vi "Get All Data Channels.vi"(8 "error in (no error)":errorcluster, 10 "framework configuration in":T1, 11 "VeriStand Data Sharing Framework in":refnum<class "VeriStand DSF.lvclass">) -> (0 "error out":errorcluster, 2 "data channel offsets":u64[](array[numeric]) format="%.0x", 3 "VeriStand Data Sharing Framework out":refnum<class "VeriStand DSF.lvclass">)   [LabVIEW 2017, in "DSF Engine.lvlib" / "VeriStand DSF.lvclass"]
uses:
  VeriStand DSF.lvclass
  DSF Core.lvlibp/Typedefs/DSF Engine Framework Configuration.ctl
  DSF Core.lvlibp/Typedefs/DSF Engine Plugin Configuration.ctl
  DSF Core.lvlibp/Typedefs/DSF Timing Info.ctl
  DSF Core.lvlibp/Typedefs/DSF Engine Plugin Thread Configuration.ctl
  DSF Core.lvlibp/Typedefs/DSF Settings Info.ctl
  DSF Core.lvlibp/Typedefs/DSF Engine Transfer Group Configuration.ctl
  DSF Core.lvlibp/Typedefs/DSF Direction.ctl
  DSF Core.lvlibp/Typedefs/DSF Engine Transfer Configuration.ctl
  DSF Core.lvlibp/Typedefs/DSF Byte Order.ctl
  DSF Core.lvlibp/Typedefs/DSF Engine Channel Configuration.ctl
  DSF Core.lvlibp/Typedefs/DSF Data Type.ctl
  DSF Core.lvlibp/Typedefs/DSF Timeout Behavior.ctl
  VeriStand DSF.lvclass/VeriStand DSF.ctl
  <vilib>/NI Veristand/Custom Device API/Data Access Type.ctl
  DSF Core.lvlibp/Classes/Configuration/Channel Count (Transfer).vi
  <vilib>/NI Veristand/Custom Device API/Custom Device API.lvlib
  DSF Core.lvlibp
  DSF Core.lvlibp/Classes/Configuration/Configuration Session.lvclass
  Shared/DSF Shared.lvlib
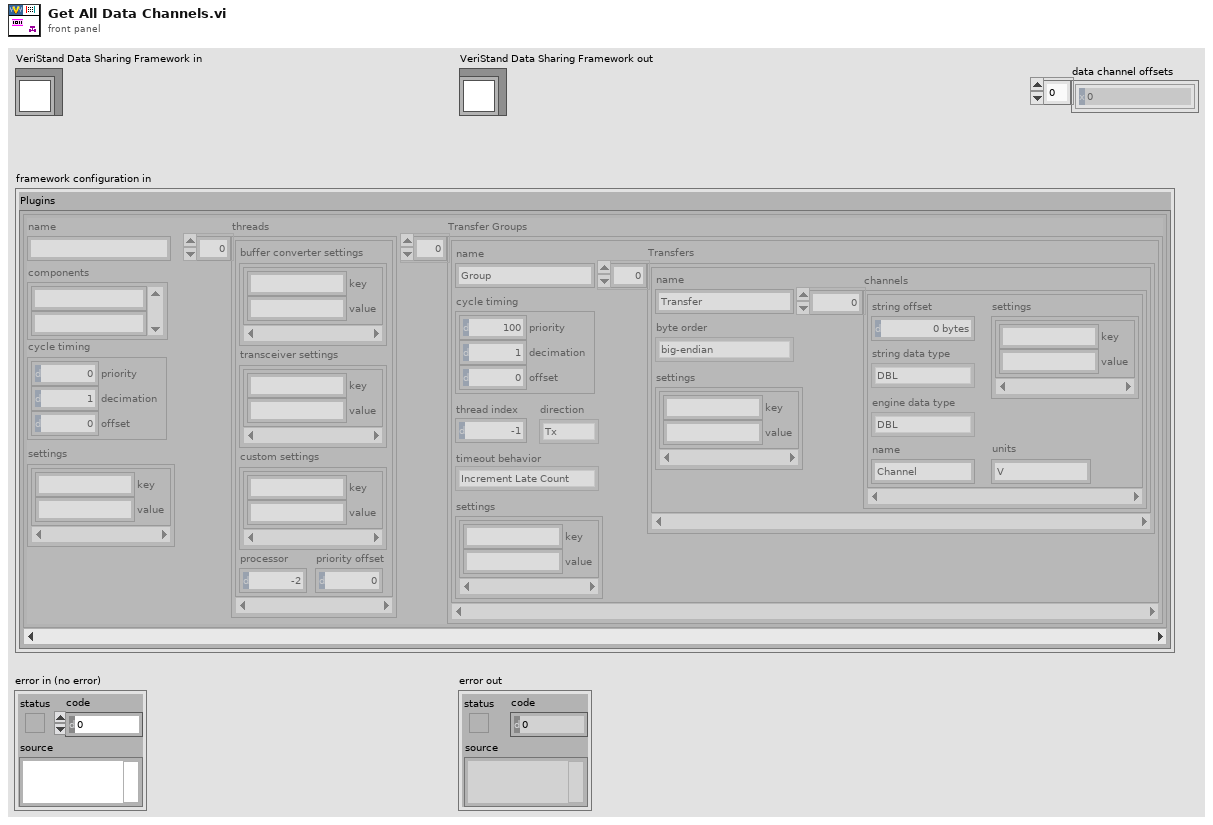
[diagram p1: front panel]
types:
  T1 = typedef "DSF Core.lvlibp/DSF Engine Framework Configuration.ctl" = cluster{"Plugins":T2[]}
  T2 = typedef "DSF Core.lvlibp/DSF Engine Plugin Configuration.ctl" = cluster{"name":string, "components":string[], "cycle timing":T3, "threads":T4[], "Transfer Groups":T6[], "settings":T5}
  T3 = typedef "DSF Core.lvlibp/DSF Timing Info.ctl" = cluster{"priority":u64, "decimation":u64, "offset":u64}
  T4 = typedef "DSF Core.lvlibp/DSF Engine Plugin Thread Configuration.ctl" = cluster{"buffer converter settings":T5, "transceiver settings":T5, "custom settings":T5, "processor":i32, "priority offset":i16}
  T5 = typedef "DSF Core.lvlibp/DSF Settings Info.ctl" = cluster{"key":string, "value":string}[]
  T6 = typedef "DSF Core.lvlibp/DSF Engine Transfer Group Configuration.ctl" = cluster{"name":string, "direction":T7, "cycle timing":T3, "thread index":i32, "settings":T5, "Transfers":T8[], "timeout behavior":T12}
  T7 = typedef "DSF Core.lvlibp/DSF Direction.ctl" = enum8{"Tx", "Rx"}
  T8 = typedef "DSF Core.lvlibp/DSF Engine Transfer Configuration.ctl" = cluster{"name":string, "byte order":T9, "settings":T5, "channels":T10[]}
  T9 = typedef "DSF Core.lvlibp/DSF Byte Order.ctl" = enum8{"big-endian", "little-endian"}
  T10 = typedef "DSF Core.lvlibp/DSF Engine Channel Configuration.ctl" = cluster{"string offset":u64, "string data type":T11, "engine data type":T11, "name":string, "settings":T5, "units":string}
  T11 = typedef "DSF Core.lvlibp/DSF Data Type.ctl" = enum8{"Bool", "SGL", "DBL", "I8", "I16", "I32", "I64", "U8", "U16", "U32", "U64"}
  T12 = typedef "DSF Core.lvlibp/DSF Timeout Behavior.ctl" = enum8{"Increment Late Count", "Throw Error"}
  T13 = enum16{"open", "replace", "create", "open or create", "replace or create", "replace or create with confirmation"}
  T14 = typedef "Custom Device API.lvlib/Custom Device Item Ref.ctl" = u64
  T15 = typedef "Custom Device API.lvlib/Data Access Type.ctl" = enum16{"Read", "Write"}
  T16 = typedef "Custom Device API.lvlib/Data Reference.ctl" = i32
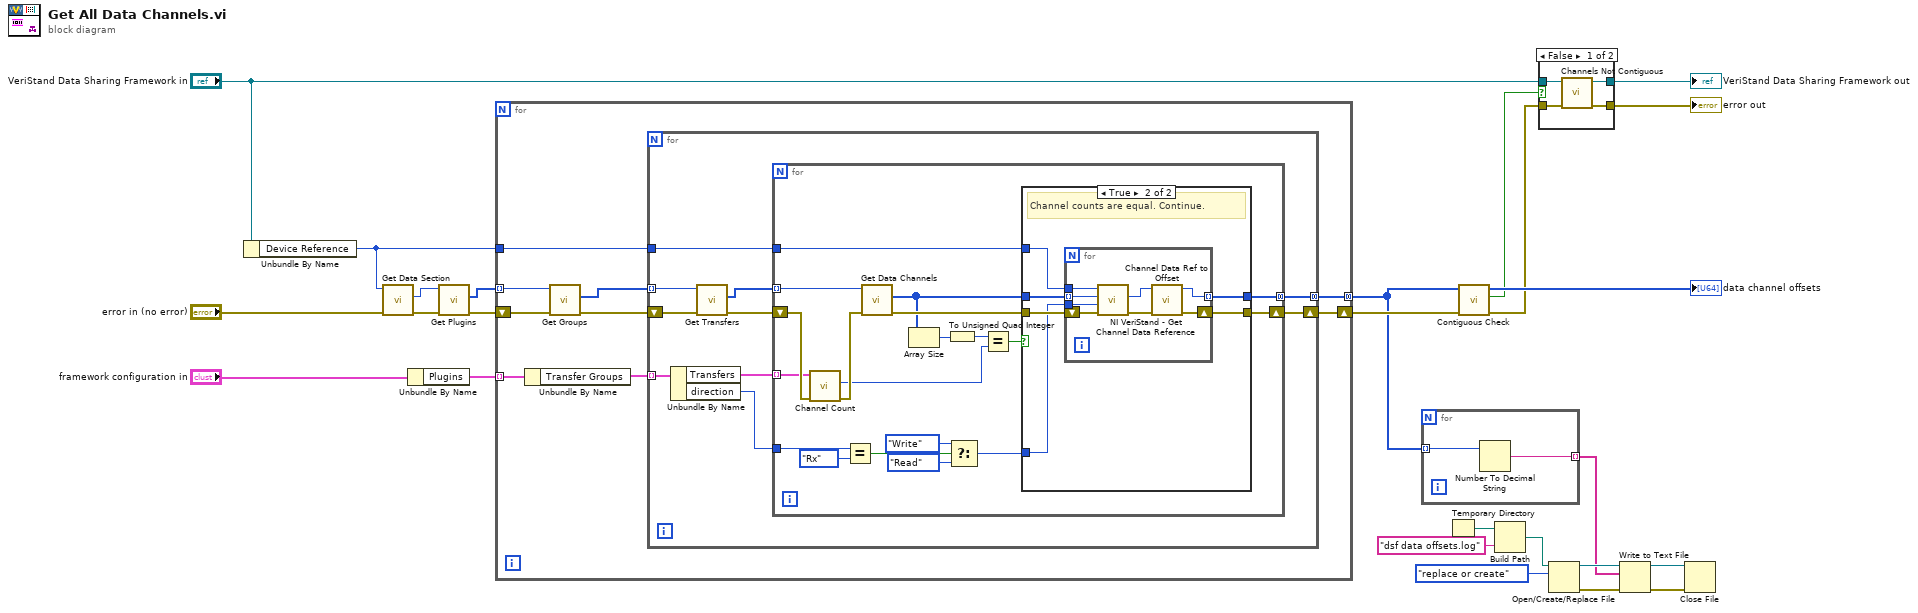
[diagram p0: block diagram]
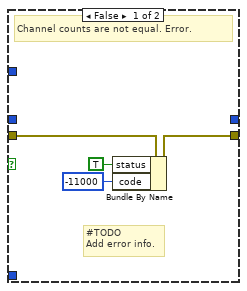
[diagram p3: hidden frame]
diagram:
  n1 = Unbundle By Name("VeriStand Data Sharing Framework in") -> ("Device Reference"=w7:T14)
  n2 = call "Get Data Section.vi"("error in (no error)"="error in (no error)", "Item Ref in"=w7) -> ("error out"=w9:errorcluster, "Data Section ref"=w8:T14)  [unwired: 6 in, 2 out]
  n3 = Unbundle By Name("framework configuration in") -> ("Plugins"=w25:T2[])
  n4 = call "Get Plugins.vi"("error in (no error)"=w9, "Item Ref in"=w8) -> ("error out"=w22:errorcluster, "Plugin refs"=w21:T14[])  [unwired: 7 in, 1 out]
  n5 = for {
    tunnel: w21 -> [w28] mode=indexing
    tunnel: w25 -> [w34] mode=indexing
    tunnel: w7 -> [w33]
    shift-right: [w32] -> w23
    shift-left: w22 -> [w29]
    tunnel: [w31] -> w12 mode=concatenating
    n6 = Unbundle By Name(w34) -> ("Transfer Groups"=w30:T6[])
    n7 = call "Get Groups.vi"("error in (no error)"=w29, "Plugin Ref in"=w28) -> ("error out"=w27:errorcluster, "Group refs"=w26:T14[])  [unwired: 7 in, 1 out]
    n8 = for {
      tunnel: w30 -> [w44] mode=indexing
      tunnel: w26 -> [w37] mode=indexing
      tunnel: w33 -> [w43]
      shift-right: [w42] -> w32
      shift-left: w27 -> [w38]
      tunnel: [w41] -> w31 mode=concatenating
      n9 = Unbundle By Name(w44) -> ("Transfers"=w40:T8[], "direction"=w39:T7)
      n10 = call "Get Transfers.vi"("error in (no error)"=w38, "Group Ref in"=w37) -> ("error out"=w36:errorcluster, "Transfer refs"=w35:T14[])  [unwired: 7 in, 1 out]
      n11 = for {
        tunnel: w40 -> [w52] mode=indexing
        tunnel: w35 -> [w48] mode=indexing
        tunnel: w39 -> [w62]
        tunnel: w43 -> [w55]
        shift-right: [w51] -> w42
        shift-left: w36 -> [w53]
        tunnel: [w50] -> w41 mode=concatenating
        n12 = call-poly "Channel Count.vi"("error in (no error)"=w53, "Transfer Configuration in"=w52) -> ("error out"=w49:errorcluster, "total channel count"=w45:u64)  [unwired: 7 in, 1 out]
        n13 = Equal?(x=w62, y=DSF_Direction."Rx") -> (x = y?=w60:bool)
        n14 = call "Get Data Channels.vi"("error in (no error)"=w49, "Transfer Ref in"=w48) -> ("error out"=w47:errorcluster, "Channels refs"=w46:T14[])  [unwired: 7 in, 1 out]
        n15 = Array Size(array=w46) -> (size(s)=w63:i32)
        n16 = To Unsigned Quad Integer(1:w63) -> (0:w56:u64)
        n17 = Select(t=Data_Access_Type."Write" ("Access"), s=w60, f=Data_Access_Type."Read") -> (s? t:f=w54:T15)
        n18 = Equal?(x=w56, y=w45) -> (x = y?=w57:bool)
        n19 = case shown="True" w57 {
          tunnel: w46 -> [_ w70]
          tunnel: w55 -> [_ w72]
          tunnel: w54 -> [_ w71]
          tunnel: w47 -> [w67 w73]
          tunnel: [w66 w68] -> w51
          tunnel: [_ w69] -> w50
          frame False {
            # "#TODO\nAdd error info."
            # "Channel counts are not equal. Error."
            n20 = Bundle By Name(cluster=w67, "status"=TRUE, "code"=-11000) -> (w66:errorcluster)
          }
          frame True {
            # "Channel counts are equal. Continue."
            n21 = for {
              tunnel: w72 -> [w80]
              tunnel: w71 -> [w79]
              tunnel: w70 -> [w78] mode=indexing
              tunnel: [w74] -> w69 mode=indexing
              shift-right: [w75] -> w68
              shift-left: w73 -> [w81]
              n22 = call <vilib>:"NI VeriStand - Get Channel Data Reference.vi"("error in (no error)"=w81, "Access"=w79, "Channel Ref in"=w78, "Device Ref in"=w80) -> ("error out"=w77:errorcluster, "Channel Data Reference"=w76:T16)  [unwired: 5 in, 1 out]
              n23 = call "Channel Data Ref to Offset.vi"("error in (no error)"=w77, "Channel Data Reference"=w76) -> ("error out"=w75:errorcluster, "channel offset"=w74:u64)  [unwired: 8 in]
            }
          }
        }
      }
    }
  }
  n24 = for {
    tunnel: w12 -> [w83] mode=indexing
    tunnel: [w82] -> w11 mode=indexing
    n25 = Number To Decimal String(number=w83) -> (decimal integer string=w82:string)  [unwired: 1 in]
  }
  n26 = Temporary Directory() -> (w19:path)
  n27 = call "Contiguous Check.vi"("error in (no error)"=w23, "channel offsets in"=w12) -> ("error out"=w3:errorcluster, "contiguous?"=w1:bool, "channel offsets out"=→"data channel offsets":u64[])  [unwired: 7 in]
  n28 = Build Path(base path=w19, name or relative path="dsf data offsets.log") -> (appended path=w17:path)
  n29 = case shown="False" w1 {
    tunnel: "VeriStand Data Sharing Framework in" -> [w87 w89]
    tunnel: [w86 w89] -> w4
    tunnel: [w85 w88] -> w2
    tunnel: w3 -> [w84 w88]
    frame False {
      n30 = call "Channels Not Contiguous.vi"("error in (no error)"=w84, "VeriStand DSF in"=w87) -> ("error out"=w85:errorcluster, "VeriStand DSF out"=w86:refnum<class "VeriStand DSF.lvclass">)  [unwired: 8 in]
    }
    frame True {
    }
  }
  "error out" <- w2
  "VeriStand Data Sharing Framework out" <- w4
  n31 = Open/Create/Replace File(file path (use dialog)=w17, operation (0:open)=T13."replace or create") -> (refnum out=w16:refnum<file>, error out=w15:errorcluster)  [unwired: 4 in, 1 out]
  n32 = Write to Text File(file (use dialog)=w16, text=w11, error in=w15) -> (refnum out=w13:refnum<file>, error out=w14:errorcluster)  [unwired: 1 in, 1 out]
  n33 = Close File(refnum=w13, error in=w14) -> ()  [unwired: 2 out]
